vi "ULx Create Channel (CI-Pulse Width).vi"(0 "task in":refnum<k24>, 5 "counters":refnum<k21>, 9 "units":i32(ring) items=["Seconds", "Ticks"], 11 "error in":errorcluster, 13 "starting edge":i32(ring) items=["Rising", "Falling"]) -> (4 "task out":refnum<k24>, 15 "error out":errorcluster)   [LabVIEW 2020]
doc: "Creates channel(s) to measure the period of digital signals."
uses:
  C:/Users/William/Documents/LV 2020 builds/LeaktestDAQ/Source-v33/ULx_LV.dll
  ULx_LV.dll
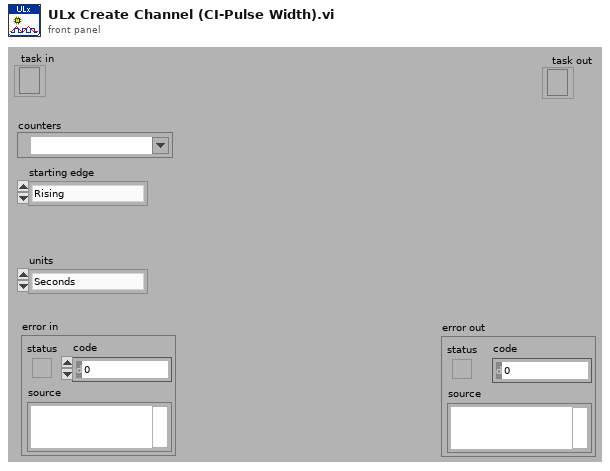
[diagram p1: front panel]
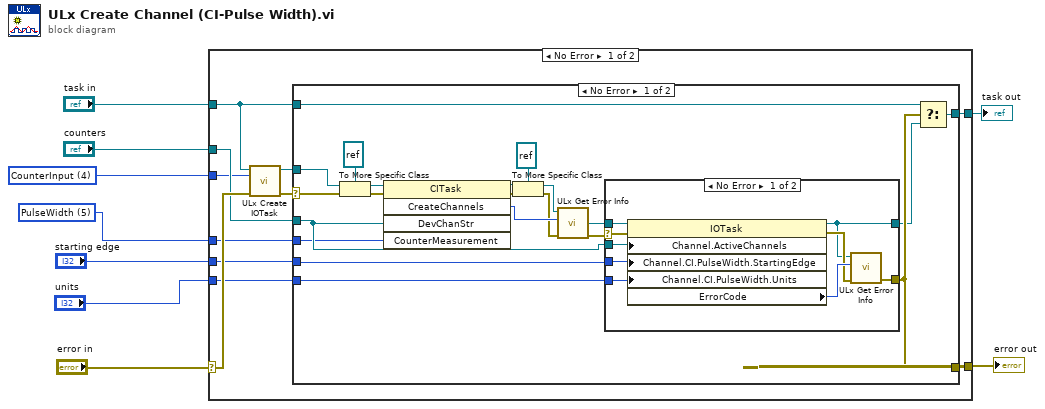
[diagram p0: block diagram]
diagram:
  w1 = 5 items=["CountEdges"=1, "Encoder"=2, "Frequency"=3, "Period"=4, "PulseWidth"=5, "Timing"=6] ("CounterMeasurement")
  w5 = 4 items=["AnalogInput", "AnalogOutput", "DigitalInput", "DigitalOutput", "CounterInput", "CounterOutput", "CompositeInput", "CompositeOutput", "TemperatureInput"] ("taskType")
  n1 = case shown="No Error" "error in" {
    selector: "error in" -> [w20 w55]
    tunnel: "task in" -> [w11 w54]
    tunnel: "counters" -> [w15 _]
    tunnel: [w18 w54] -> w7
    tunnel: [w17 w55] -> w6
    tunnel: w5 -> [w14 _]
    tunnel: "starting edge" -> [w13 _]
    tunnel: "units" -> [w12 _]
    tunnel: w1 -> [w10 _]
    frame No Error {
      n2 = call "ULx Create IOTask.vi"("error in"=w20, "taskType"=w14, "i/o task in"=w11) -> ("error out"=w19:errorcluster, "i/o task out"=w16:refnum<k24>)  [unwired: 7 in]
      n3 = case shown="No Error" w19 {
        selector: w19 -> [w38 w53]
        tunnel: [w24 w53] -> w17
        tunnel: [w25 w52] -> w18
        tunnel: w16 -> [w36 _]
        tunnel: w15 -> [w33 _]
        tunnel: w13 -> [w32 _]
        tunnel: w12 -> [w31 _]
        tunnel: w11 -> [w22 w52]
        tunnel: w10 -> [w21 _]
        frame No Error {
          n4 = To More Specific Class(target class=refnum<k24> refnum, reference=w36, error in=w38) -> (specific class reference=w39:refnum<k24>, error out=w37:errorcluster)
          n5 = invoke class="CITask" method="CreateChannels"(reference=w39, error in=w37, "DevChanStr"=w33, "CounterMeasurement"=w21) -> (reference out=w29:refnum<k24>, error out=w28:errorcluster, "CreateChannels"=w35:i32)  [unwired: 1 in, 2 out]
          n6 = To More Specific Class(target class=refnum<k24> refnum, reference=w29, error in=w28) -> (specific class reference=w26:refnum<k24>, error out=w27:errorcluster)
          n7 = call "ULx Get Error Info.vi"("error in"=w27, "ErrorCode"=w35, "task in"=w26) -> ("error out"=w34:errorcluster)  [unwired: 8 in]
          n8 = case shown="No Error" w34 {
            selector: w34 -> [w49 w51]
            tunnel: w26 -> [w48 w50]
            tunnel: w33 -> [w47 _]
            tunnel: [w44 w51] -> w24
            tunnel: w32 -> [w43 _]
            tunnel: w31 -> [w42 _]
            tunnel: [w41 w50] -> w23
            frame No Error {
              n9 = property class="IOTask"(reference=w48, error in=w49, "Channel.ActiveChannels"=w47, "Channel.CI.PulseWidth.StartingEdge"=w43, "Channel.CI.PulseWidth.Units"=w42) -> (reference out=w41:refnum<k24>, error out=w45:errorcluster, "ErrorCode"=w46:i32)
              n10 = call "ULx Get Error Info.vi"("error in"=w45, "ErrorCode"=w46, "task in"=w41) -> ("error out"=w44:errorcluster)  [unwired: 8 in]
            }
            frame Error {
            }
          }
          n11 = Select(t=w22, s=w24, f=w23) -> (s? t:f=w25:refnum<k24>)
        }
        frame Error {
        }
      }
    }
    frame Error {
    }
  }
  "error out" <- w6
  "task out" <- w7
